vi "SetParam.vi"(8 "error in (no error)":errorcluster caption="entrée d'erreur (pas d'erreur)", 10 "fetch_lfw_pairs":T1={"subset"="train", "funneled"=TRUE, "resize"=0.5, "color"=FALSE, "slice_"={"Cluster"={"height"=70, "width"=195}, "Cluster 2"={"height"=78, "width"=172}}, "download_if_missing"=TRUE, "Returns"="Data"}, 11 "lfw_pairs.lvclass":refnum<class "lfw_pairs.lvclass">) -> (0 "error out":errorcluster caption="sortie d'erreur", 3 "lfw_pairs.lvclass":refnum<class "lfw_pairs.lvclass">)   [LabVIEW 2020, in "lfw_pairs.lvclass"]
doc: "Set Parameters"
uses:
  lfw_pairs.lvclass
  lfw_pairs.lvclass/lfw_pairs.ctl
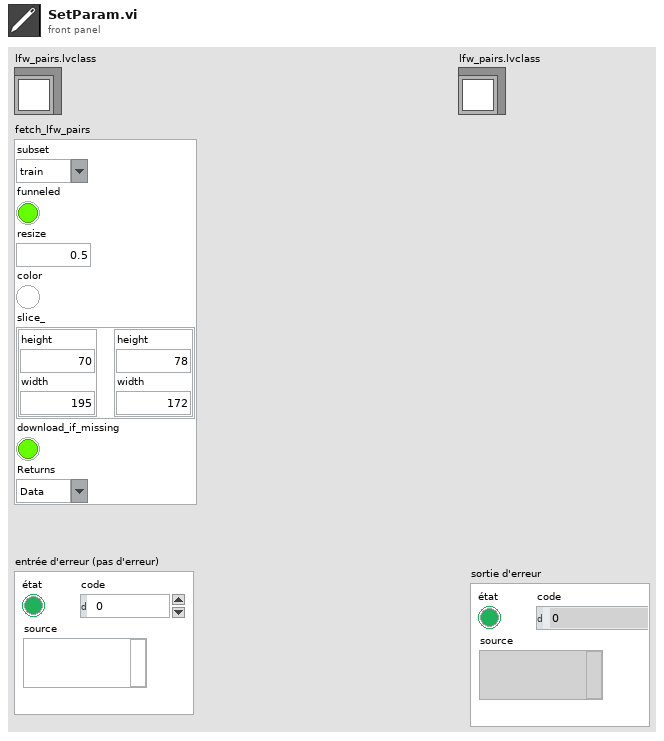
[diagram p1: front panel]
types:
  T1 = cluster{"subset":string, "funneled":bool, "resize":dbl, "color":bool, "slice_":cluster{"Cluster":cluster{"height":u32, "width":u32}, "Cluster 2":cluster{"height":u32, "width":u32}}, "download_if_missing":bool, "Returns":string}
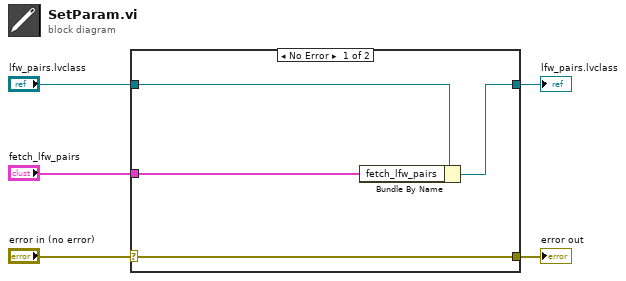
[diagram p0: block diagram]
diagram:
  n1 = case shown="No Error" "error in (no error)" {
    selector: "error in (no error)" -> [w9 w10]
    tunnel: [w9 w10] -> w4
    tunnel: [w7 w11] -> w2
    tunnel: "lfw_pairs.lvclass" -> [w8 w11]
    tunnel: "fetch_lfw_pairs" -> [w6 _]
    frame No Error {
      n2 = Bundle By Name(cluster=w8, "fetch_lfw_pairs"=w6) -> (w7:refnum<class "lfw_pairs.lvclass">)
    }
    frame Error {
    }
  }
  "error out" <- w4
  "lfw_pairs.lvclass" <- w2
